vi "CC Rd Wr Configuration obsolete.vi"(7 "Write? (F:Read)":bool, 8 "error in (no error)":errorcluster, 11 "Hardware Config":T1) -> (0 "error out":errorcluster, 3 "Hardware Config out":T1)   [LabVIEW 2019]
uses:
  typedefs/CC cluster Hardware Config.ctl
  1f939ea0-859f-4775-b814-4454fe913132.vi
  30e832c1-cc5b-4690-af76-45f6ccf45904.vi
  348af09c-8964-40b0-b908-ca05888150ef.vi
  <vilib>/JDP Science/JSONtext/JSON text to Variant.vi
  <vilib>/JDP Science/JSONtext/Variant to JSON Text.vi
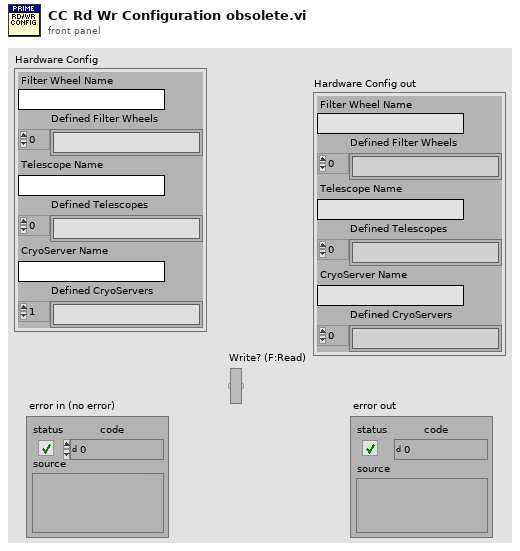
[diagram p1: front panel]
types:
  T1 = typedef "CC cluster Hardware Config.ctl" = cluster{"Filter Wheel Name":string, "Defined Filter Wheels":string[], "Telescope Name":string, "Defined Telescopes":string[], "CryoServer Name":string, "Defined CryoServers":string[]}
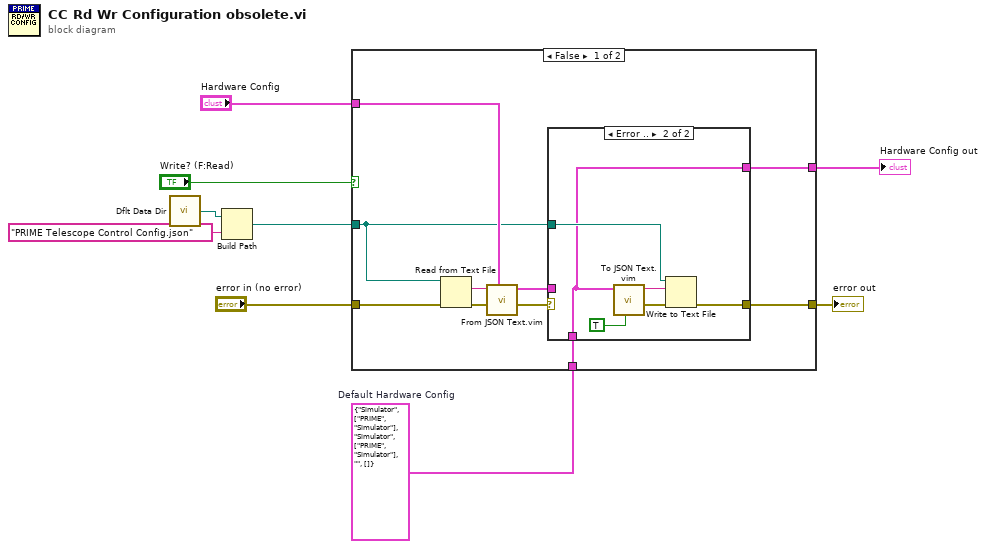
[diagram p0: block diagram]
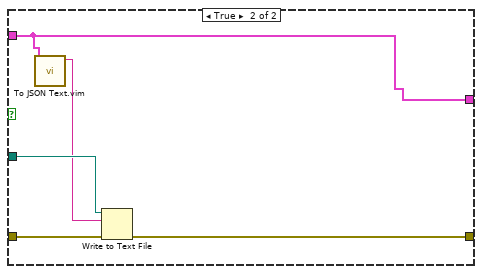
[diagram p3: hidden frame]
diagram:
  w1 = T1 {"Filter Wheel Name"="Simulator", "Defined Filter Wheels"=["PRIME", "Simulator"], "Telescope Name"="Simulator", "Defined Telescopes"=["PRIME", "Simulator"], "CryoServer Name"="", "Defined CryoServers"=[]}  # Default Hardware Config
  n1 = call <vilib>:"Dflt Data Dir.vi"() -> ("App:Default Data Directory"=w8:path)
  n2 = Build Path(base path=w8, name or relative path="PRIME Telescope Control Config.json") -> (appended path=w6:path)
  n3 = case shown="False" "Write? (F:Read)" {
    tunnel: "error in (no error)" -> [w19 w32]
    tunnel: w6 -> [w11 w31]
    tunnel: "Hardware Config" -> [w18 w28]
    tunnel: [w10 w29] -> w3
    tunnel: [w13 w28] -> w2
    tunnel: w1 -> [w12 _]
    frame False {
      n4 = Read from Text File(file (use dialog)=w11, error in=w19) -> (text=w17:string, error out=w16:errorcluster)  [unwired: 2 in, 2 out]
      n5 = call "From JSON Text.vim"("Data Type and Default Value"=w18, "error in (no error)"=w16, "JSON"=w17) -> ("error out"=w15:errorcluster, "Data out"=w14:T1)  [unwired: 7 in]
      n6 = case shown="Error .." w15 {
        selector: w15 -> [w20 _]
        tunnel: w14 -> [w21 _]
        tunnel: [w21 w23] -> w13
        tunnel: w12 -> [_ w23]
        tunnel: w11 -> [_ w24]
        tunnel: [w20 w22] -> w10
        frame No Error {
        }
        frame Error {
          n7 = call "To JSON Text.vim"("Pretty Print?"=TRUE, "Anything"=w23) -> ("error out"=w27:errorcluster, "<JSON>"=w25:string)  [unwired: 8 in]
          n8 = Write to Text File(file (use dialog)=w24, text=w25, error in=w27) -> (error out=w22:errorcluster)  [unwired: 1 in, 2 out]
        }
      }
    }
    frame True {
      n9 = call "To JSON Text.vim"("Anything"=w28) -> ("<JSON>"=w30:string)  [unwired: 9 in, 1 out]
      n10 = Write to Text File(file (use dialog)=w31, text=w30, error in=w32) -> (error out=w29:errorcluster)  [unwired: 1 in, 2 out]
    }
  }
  "error out" <- w3
  "Hardware Config out" <- w2
